vi "direct_ads_vol_dw_dT_pTpsatRho.vi"(0 "WorkingPair (Input)":T1={"no_iso"=1, "no_p_sat"=1, "path_db"="D:\\Driesel\\SorpLibLocal\\LabVIEW_wrapper\\data\\json\\sorpproplib_minimalExample.json", "wp_as"="silicagel", "wp_st"="123", "wp_iso"="DubininArctan1", "wp_rf"="water", "rf_rhol"="SaturatedLiquidDensity_EoS1", "no_rhol"=1, "rf_psat"="VaporPressure_EoS1"}, 1 "Saturation pressure in Pa (Input)":dbl, 2 "Temperature in K (Input)":dbl, 3 "Pressure Pa (Input)":dbl, 5 "Der. of saturation pressure wrt. temperature in Pa/K (Input)":dbl, 7 "Density of adsorpt in kg/m3 (Input)":dbl, 9 "Der. of density of adsorpt wrt. temperature in kg/m3/K (Input)":dbl, 11 "Error (Input)":errorcluster) -> (4 "Der. of loading wrt. temperature in kg/kg/K (Output)":dbl, 15 "Error (Output)":errorcluster caption="Error(Output)")   [LabVIEW 2017]
doc: "direct_ads_vol_dw_dT_pTpsatRho:\n * -------------------------------\n *\n * Calculates derivative of equilibrium loading dw_dp with respect to\n * temperature in kg/kg/K depending on equilibrium pressure p in Pa, equilibrium\n * temperature T in K, saturation pressure p_Sat in Pa, density of adsorpt\n * rho in kg/m³, derivative of saturation pressure with respect to temperature\n * dp_sat_dT in Pa/K and derivative of density of adsorpt with respect to\n * temperature drho_dT in kg/m³/K.\n *\n * Parameters:\n * -----------\n * double p_Pa:\n * Equilibrium pressure in Pa.\n * double T_K:\n * Equilibrium temperature in K.\n * double p_sat_Pa:\n * Saturation pressure in Pa.\n * double rho_kgm3:\n * Density of adsorpt in kg/m³.\n * double dp_sat_dT_PaK:\n * Derivative of saturation pressure wrt. temperature in Pa/K.\n * double drho_dT_kgm3K:\n * Derivative of density of adsorpt wrt. temperature in kg/m³/K.\n *\n * const char *path_db:\n * Path to database.\n * const char *wp_as:\n * Name of sorbent.\n * const char *wp_st:\n * Name of sub-type of sorbent.\n * const char *wp_rf:\n * Name of refrigerant.\n * const char *wp_iso:\n * Name of isotherm.\n * int no_iso:\n * ID of isotherm (i.e. when more than one isotherm is available)\n * const char *rf_psat:\n * Name of calculation approach for vapor pressure.\n * int no_p_sat:\n * ID of vapor pressure equation (i.e. when more than one equation is\n * available)\n * const char *rf_rhol:\n * Name of calculation approach for liquid density.\n * int no_rhol:\n * ID of liquid density equation (i.e. when more than one equation is\n * available)\n *\n * Returns:\n * --------\n * double:\n * Derivative of equilibrium loading wrt. temperature in kg/kg/K.\n *\n * Remarks:\n * --------\n * This function is only valid for isotherm models based on the volumetric\n * approach.\n *\n * History:\n * --------\n * 07/07/2021, by Jannik Driesel (supervised by Mirko Engelpracht):\n * First implementation."
uses:
  data/win32bit/libsorpPropLib.dll
panel:
  # "Path to database"
  # "Name of sorbent"
  # "Name of sub-type of sorbent"
  # "Name of refrigerant"
  # "Name of isotherm"
  # "ID of isotherm"
  # "Name of calculation approach for vapor pressure"
  # "ID of vapor pressure equation"
  # "Name of calculation approach for liquid density"
  # "ID of liquid density equation"
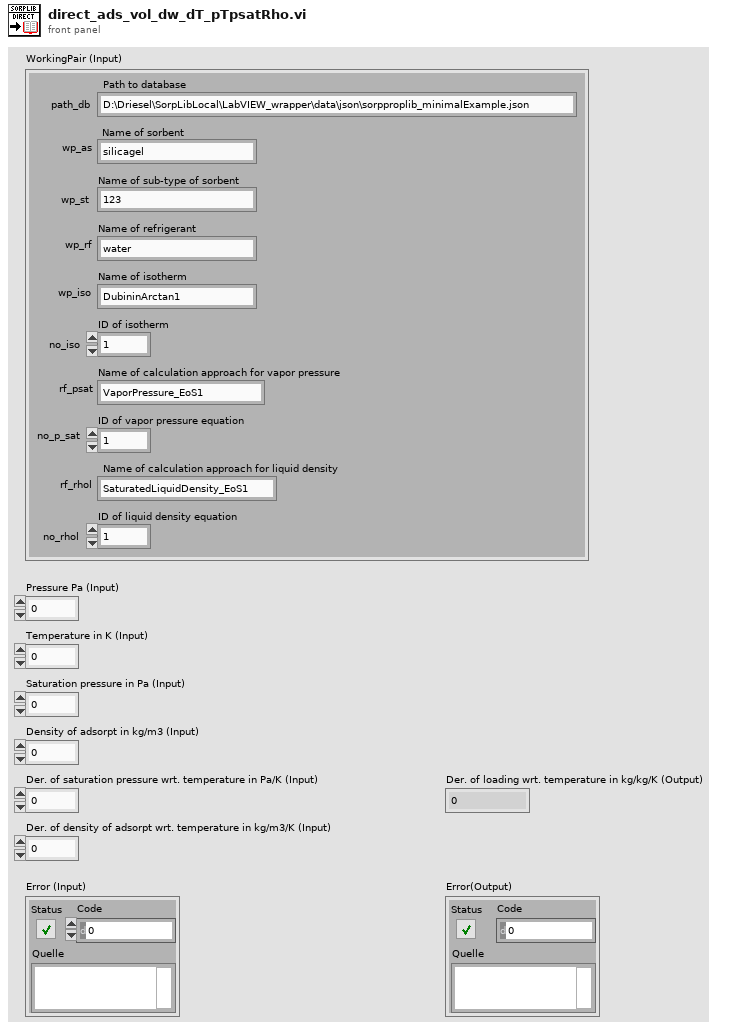
[diagram p1: front panel]
types:
  T1 = cluster{"no_iso":i32, "no_p_sat":i32, "path_db":string, "wp_as":string, "wp_st":string, "wp_iso":string, "wp_rf":string, "rf_rhol":string, "no_rhol":i32, "rf_psat":string}
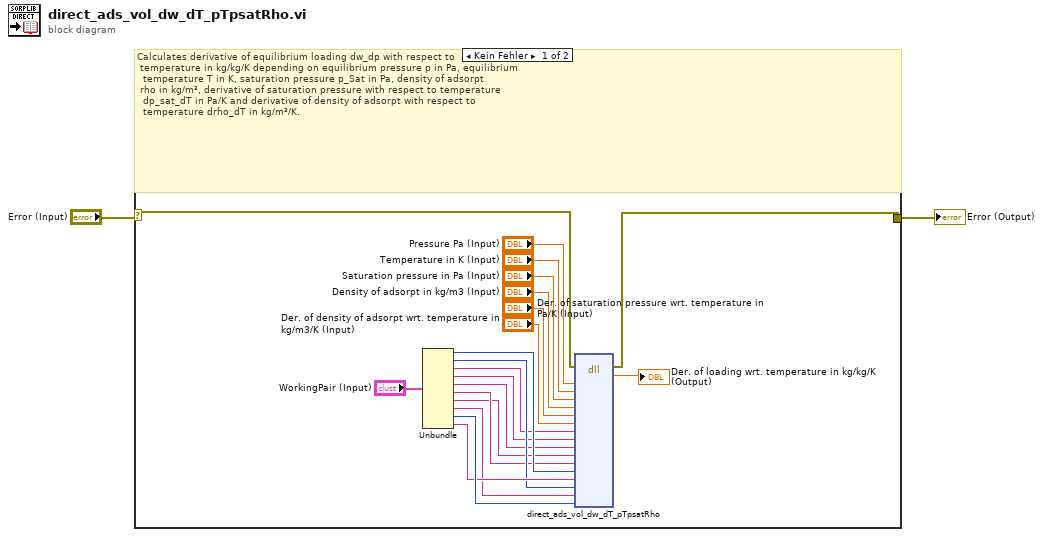
[diagram p0: block diagram]
diagram:
  n1 = case shown="Kein Fehler" "Error (Input)" {
    selector: "Error (Input)" -> [w10 w23]
    tunnel: [w9 w23] -> w1
    frame No Error {
      # "Calculates derivative of equilibrium loading dw_dp with respect to\n temperature in kg/kg/K depending on equilibrium pressure p in Pa, equilibrium\n  temperature T in K, saturation pressure p_Sat in Pa, density of adsorpt\n rho in kg/m³, derivative of saturation pressure with respect to temperature\n  dp_sat_dT in Pa/K and derivative of density of adsorpt with respect to\n  temperature drho_dT in kg/m³/K."
      n2 = Unbundle("WorkingPair (Input)") -> ("no_iso"=w18:i32, "no_p_sat"=w19:i32, "path_db"=w12:string, "wp_as"=w13:string, "wp_st"=w14:string, "wp_iso"=w16:string, "wp_rf"=w15:string, "rf_rhol"=w17:string, "no_rhol"=w21:i32, "rf_psat"=w20:string)
      n3 = dll-call lib="D:/Driesel/SorpLibLocal/LabVIEW_wrapper/data/win32bit/libsorpPropLib.dll" fn="direct_ads_vol_dw_dT_pTpsatRho"(error in=w10, "p_Pa"="Pressure Pa (Input)", "T_K"="Temperature in K (Input)", "p_sat_Pa"="Saturation pressure in Pa (Input)", "rho_kgm3"="Density of adsorpt in kg/m3 (Input)", "dp_sat_dT_PaK"="Der. of saturation pressure wrt. temperature in Pa/K (Input)", "drho_dT_kgm3K"="Der. of density of adsorpt wrt. temperature in kg/m3/K (Input)", "path_db"=w12, "wp_as"=w13, "wp_st"=w14, "wp_rf"=w15, "wp_iso"=w16, "no_iso"=w18, "rf_psat"=w20, "no_p_sat"=w19, "rf_rhol"=w17, "no_rhol"=w21) -> (error out=w9:errorcluster, "dw_dT_kgkgK"=→"Der. of loading wrt. temperature in kg/kg/K (Output)":dbl)  [unwired: 18 in, 1 out]
    }
    frame Error {
      # "Error - No calculations"
    }
  }
  "Error (Output)" <- w1
